vi "REQ-REP.vi"() -> ()   [LabVIEW 2018]
uses:
  RxTx/CM_RxTx.lvclass
  socket REQ/socket REQ.lvclass
  C:/Users/Denis/Desktop/communication-manager/communication-manager/Socket/Socket.lvclass
  socket REP/socket REP.lvclass
  Socket/Socket.lvclass
  <vilib>/addons/zeromq/zmq_context.lvclass
panel:
  in  "config file folder":path=path "C:/Users/Denis/Desktop/communication-manager/communication-manager/CFG file"
  in  "socket REP.lvclass":refnum<class "socket REP.lvclass">
  in  "socket REQ.lvclass":refnum<class "socket REQ.lvclass">
  out "error out 3":errorcluster
  in  "Queue RX 2":refnum<class "CM_RxTx.lvclass">
  out "Received message":string
  out "error out 2":errorcluster
  in  "Queue RX":refnum<class "CM_RxTx.lvclass">
  in  "stop":bool
  in  "message":string
  in  "send":bool
  # "REQ endpoint"
  # "REP endpoint"
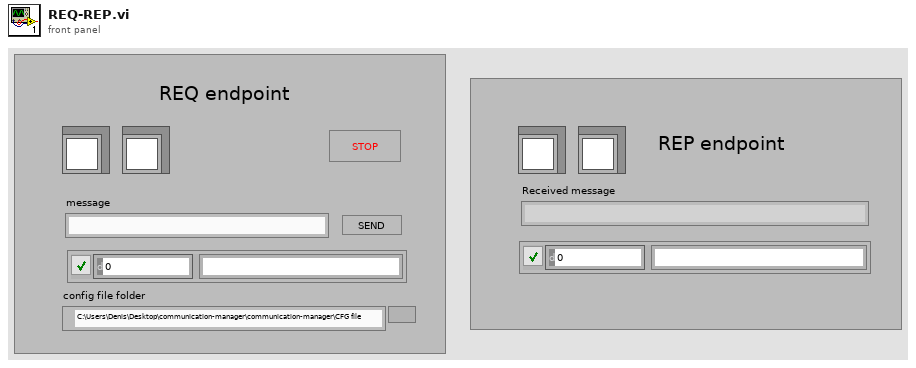
[diagram p1: front panel]
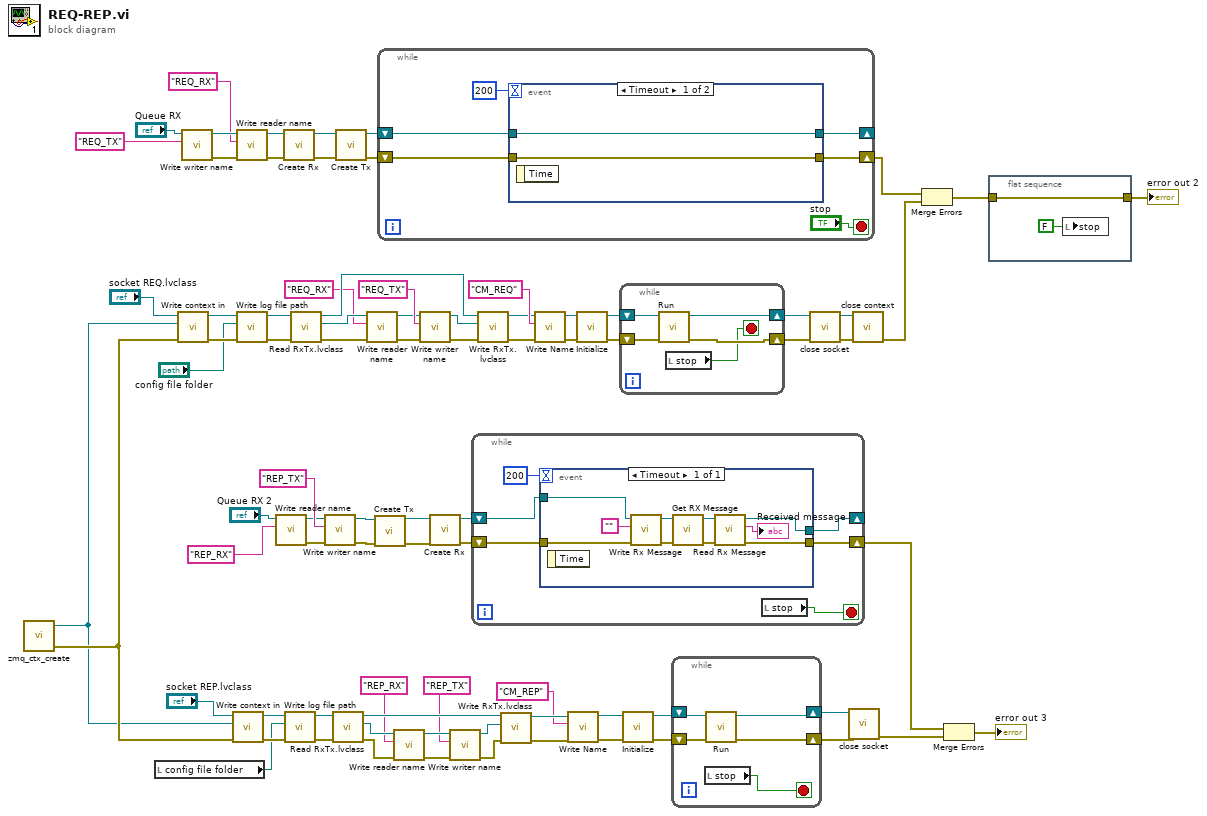
[diagram p0: block diagram]
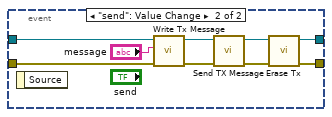
[diagram p2: hidden frame]
diagram:
  n1 = call <vilib>:"zmq_ctx_create.vi"() -> ("error out"=w41:errorcluster, "context out"=w40:refnum<class "zmq_context.lvclass">)  [unwired: 4 in]
  n2 = local read "config file folder"() -> (w1:path)
  n3 = call-dynamic "Write context in.vi"("error in (no error)"=w41, "zeromq.lvlib:ZeroMQ Context"=w40, "Socket in"="socket REQ.lvclass") -> ("error out"=w6:errorcluster, "Socket out"=w4:refnum<class "socket REQ.lvclass">)  [unwired: 7 in]
  n4 = call-dynamic "Write writer name.vi"("Tx name"="REQ_TX", "RxTx in"="Queue RX") -> ("error out"=w24:errorcluster, "RxTx out"=w23:refnum<class "CM_RxTx.lvclass">)  [unwired: 8 in]
  n5 = call-dynamic "Write context in.vi"("error in (no error)"=w41, "zeromq.lvlib:ZeroMQ Context"=w40, "Socket in"="socket REP.lvclass") -> ("error out"=w7:errorcluster, "Socket out"=w10:refnum<class "socket REP.lvclass">)  [unwired: 7 in]
  n6 = call-dynamic "Write reader name.vi"("error in (no error)"=w24, "RX name"="REQ_RX" ("Tx name"), "RxTx in"=w23) -> ("error out"=w26:errorcluster, "RxTx out"=w25:refnum<class "CM_RxTx.lvclass">)  [unwired: 7 in]
  n7 = call-dynamic "Write log file path.vi"("error in (no error)"=w6, "log file path"="config file folder", "Socket in"=w4) -> ("error out"=w5:errorcluster, "Socket out"=w3:refnum<class "socket REQ.lvclass">)  [unwired: 7 in]
  n8 = call-dynamic "Write reader name.vi"("RX name"="REP_RX" ("string"), "RxTx in"="Queue RX 2") -> ("error out"=w17:errorcluster, "RxTx out"=w14:refnum<class "CM_RxTx.lvclass">)  [unwired: 8 in]
  n9 = call "Create Rx.vi"("error in (no error)"=w26, "RxTx in"=w25) -> ("error out"=w28:errorcluster, "RxTx out"=w27:refnum<class "CM_RxTx.lvclass">)  [unwired: 8 in]
  n10 = call-dynamic "Write log file path.vi"("error in (no error)"=w7, "log file path"=w1, "Socket in"=w10) -> ("error out"=w8:errorcluster, "Socket out"=w9:refnum<class "socket REP.lvclass">)  [unwired: 7 in]
  n11 = call-dynamic "Read RxTx.lvclass.vi"("error in (no error)"=w5, "Socket in"=w3) -> ("error out"=w70:errorcluster, "RxTx.lvclass"=w74:refnum<class "CM_RxTx.lvclass">, "Socket out"=w71:refnum<class "socket REQ.lvclass">)  [unwired: 7 in]
  n12 = call-dynamic "Write writer name.vi"("error in (no error)"=w17, "Tx name"="REP_TX" ("string"), "RxTx in"=w14) -> ("error out"=w16:errorcluster, "RxTx out"=w15:refnum<class "CM_RxTx.lvclass">)  [unwired: 7 in]
  n13 = call-dynamic "Read RxTx.lvclass.vi"("error in (no error)"=w8, "Socket in"=w9) -> ("error out"=w50:errorcluster, "RxTx.lvclass"=w46:refnum<class "CM_RxTx.lvclass">, "Socket out"=w49:refnum<class "socket REP.lvclass">)  [unwired: 7 in]
  n14 = call "Create Tx.vi"("error in (no error)"=w28, "RxTx in"=w27) -> ("error out"=w79:errorcluster, "RxTx out"=w81:refnum<class "CM_RxTx.lvclass">)  [unwired: 8 in]
  n15 = call-dynamic "Write reader name.vi"("error in (no error)"=w70, "RX name"="REQ_RX" ("reader name"), "RxTx in"=w74) -> ("error out"=w69:errorcluster, "RxTx out"=w73:refnum<class "CM_RxTx.lvclass">)  [unwired: 7 in]
  n16 = call "Create Tx.vi"("error in (no error)"=w16, "RxTx in"=w15) -> ("error out"=w18:errorcluster, "RxTx out"=w19:refnum<class "CM_RxTx.lvclass">)  [unwired: 8 in]
  n17 = while {
    shift-right: [w84] -> _
    shift-left: w81 -> [w86]
    shift-right: [w83] -> w57
    shift-left: w79 -> [w85]
    stop <- "stop" stop-if-true
    n18 = event shown="[0] Timeout" {
      selector: _ -> [_ _]
      dyn-events: _ -> [_ _]
      timeout: 200 -> [_ _]
      tunnel: [w89 w95] -> w84
      tunnel: [w88 w94] -> w83
      tunnel: w86 -> [w89 w91]
      tunnel: w85 -> [w88 w90]
      event Timeout {
        n19 = event-data() -> ()  [unwired: 1 in, 1 out]
      }
      event "send": Value Change {
        n20 = event-data() -> ()  [unwired: 1 in, 1 out]
        n21 = call "Write Tx Message.vi"("error in (no error)"=w90, "Tx Message"="message", "RxTx in"=w91) -> ("error out"=w92:errorcluster, "RxTx out"=w97:refnum<class "CM_RxTx.lvclass">)  [unwired: 7 in]
        n22 = call "Send TX Message.vi"("error in (no error)"=w92, "RxTx in"=w97) -> ("error out"=w93:errorcluster, "RxTx out"=w96:refnum<class "CM_RxTx.lvclass">)  [unwired: 8 in]
        n23 = call "Erase Tx.vi"("error in (no error)"=w93, "RxTx in"=w96) -> ("error out"=w94:errorcluster, "RxTx out"=w95:refnum<class "CM_RxTx.lvclass">)  [unwired: 8 in]
      }
    }
  }
  n24 = call-dynamic "Write reader name.vi"("error in (no error)"=w50, "RX name"="REP_RX" ("reader name"), "RxTx in"=w46) -> ("error out"=w51:errorcluster, "RxTx out"=w47:refnum<class "CM_RxTx.lvclass">)  [unwired: 7 in]
  n25 = call-dynamic "Write writer name.vi"("error in (no error)"=w69, "Tx name"="REQ_TX" ("writer name"), "RxTx in"=w73) -> ("error out"=w68:errorcluster, "RxTx out"=w72:refnum<class "CM_RxTx.lvclass">)  [unwired: 7 in]
  n26 = call "Create Rx.vi"("error in (no error)"=w18, "RxTx in"=w19) -> ("error out"=w34:errorcluster, "RxTx out"=w35:refnum<class "CM_RxTx.lvclass">)  [unwired: 8 in]
  n27 = call-dynamic "Write writer name.vi"("error in (no error)"=w51, "Tx name"="REP_TX" ("writer name"), "RxTx in"=w47) -> ("error out"=w52:errorcluster, "RxTx out"=w48:refnum<class "CM_RxTx.lvclass">)  [unwired: 7 in]
  n28 = while {
    shift-right: [w102] -> _
    shift-left: w35 -> [w103]
    shift-right: [w100] -> w32
    shift-left: w34 -> [w101]
    stop <- w99 stop-if-true
    n29 = event shown="[0] Timeout" {
      selector: _ -> [_]
      dyn-events: _ -> [_]
      timeout: 200 -> [_]
      tunnel: w103 -> [w111]
      tunnel: [w109] -> w102
      tunnel: w101 -> [w106]
      tunnel: [w105] -> w100
      event Timeout {
        n30 = event-data() -> ()  [unwired: 1 in, 1 out]
        n31 = call "Write Rx Message.vi"("error in (no error)"=w106, "Rx Message"="", "RxTx in"=w111) -> ("error out"=w108:errorcluster, "RxTx out"=w110:refnum<class "CM_RxTx.lvclass">)  [unwired: 7 in]
        n32 = call "Get RX Message.vi"("error in (no error)"=w108, "RxTx in"=w110) -> ("error out"=w112:errorcluster, "RxTx out"=w114:refnum<class "CM_RxTx.lvclass">)  [unwired: 7 in, 1 out]
        n33 = call "Read Rx Message.vi"("error in (no error)"=w112, "RxTx in"=w114) -> ("error out"=w105:errorcluster, "Rx Message"=→"Received message":string, "RxTx out"=w109:refnum<class "CM_RxTx.lvclass">)  [unwired: 7 in]
      }
    }
    n34 = local read "stop"() -> (w99:bool)
  }
  n35 = call-dynamic "Write RxTx.lvclass.vi"("error in (no error)"=w68, "RxTx.lvclass"=w72, "Socket in"=w71) -> ("error out"=w58:errorcluster, "Socket out"=w59:refnum<class "socket REQ.lvclass">)  [unwired: 7 in]
  n36 = call-dynamic "Write RxTx.lvclass.vi"("error in (no error)"=w52, "RxTx.lvclass"=w48, "Socket in"=w49) -> ("error out"=w55:errorcluster, "Socket out"=w54:refnum<class "socket REP.lvclass">)  [unwired: 7 in]
  n37 = call-dynamic "Write Name.vi"("error in (no error)"=w58, "Name"="CM_REQ", "Socket in"=w59) -> ("error out"=w66:errorcluster, "Socket out"=w67:refnum<class "socket REQ.lvclass">)  [unwired: 7 in]
  n38 = call-dynamic "Write Name.vi"("error in (no error)"=w55, "Name"="CM_REP", "Socket in"=w54) -> ("error out"=w42:errorcluster, "Socket out"=w43:refnum<class "socket REP.lvclass">)  [unwired: 7 in]
  n39 = call-dynamic "Initialize.vi"("error in (no error)"=w66, "socket REQ in"=w67) -> ("error out"=w63:errorcluster, "socket REQ out"=w65:refnum<class "socket REQ.lvclass">)  [unwired: 8 in]
  n40 = while {
    shift-right: [w117] -> w64
    shift-left: w65 -> [w119]
    shift-right: [w116] -> w62
    shift-left: w63 -> [w118]
    stop <- w115 stop-if-true
    n41 = call-dynamic "Run.vi"("error in (no error)"=w118, "socket REQ in"=w119) -> ("error out"=w116:errorcluster, "socket REQ out"=w117:refnum<class "socket REQ.lvclass">)  [unwired: 8 in]
    n42 = local read "stop"() -> (w115:bool)
  }
  n43 = call-dynamic "Initialize.vi"("error in (no error)"=w42, "socket REP in"=w43) -> ("error out"=w38:errorcluster, "socket REP out"=w39:refnum<class "socket REP.lvclass">)  [unwired: 8 in]
  n44 = while {
    shift-right: [w122] -> w36
    shift-left: w39 -> [w124]
    shift-right: [w121] -> w37
    shift-left: w38 -> [w123]
    stop <- w120 stop-if-true
    n45 = local read "stop"() -> (w120:bool)
    n46 = call-dynamic "Run.vi"("error in (no error)"=w123, "socket REP in"=w124) -> ("error out"=w121:errorcluster, "socket REP out"=w122:refnum<class "socket REP.lvclass">)  [unwired: 8 in]
  }
  n47 = call "close socket.vi"("error in (no error)"=w62, "Socket in"=w64) -> ("error out"=w77:errorcluster, "Socket out"=w76:refnum<class "socket REQ.lvclass">)  [unwired: 8 in]
  n48 = call "close socket.vi"("error in (no error)"=w37, "Socket in"=w36) -> ("error out"=w31:errorcluster)  [unwired: 8 in, 1 out]
  n49 = call-dynamic "close context.vi"("error in (no error)"=w77, "Socket in"=w76) -> ("error out"=w56:errorcluster)  [unwired: 8 in, 1 out]
  n50 = Merge Errors(w57, w56) -> (w12:errorcluster)
  n51 = Merge Errors(w32, w31) -> (→"error out 3":errorcluster)
  n52 = flat-sequence {
    tunnel: w12 -> [w126]
    tunnel: [w126] -> w11
    frame #0 {
      n53 = local write "stop"(FALSE ("stop")) -> ()
    }
  }
  "error out 2" <- w11
